vi "Load Config.vi"(11 "Config Path":path) -> (1 "Twitter":cluster{"Enabled":bool, "Tag":string}, 2 "Flickr":T2, 3 "Photobooth":T1)   [LabVIEW 2012]
uses:
  <vilib>/Utility/config.llb/NI_LVConfig.lvlib
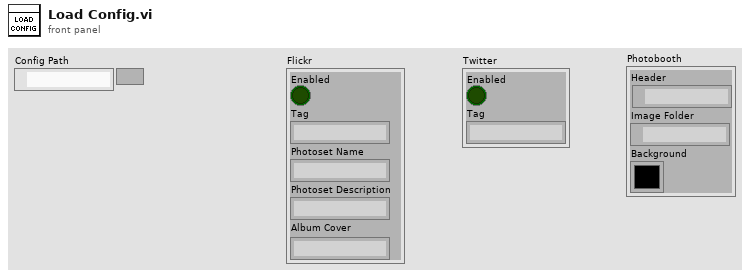
[diagram p1: front panel]
types:
  T1 = cluster{"Header":path, "Image Folder":path, "Background":u32}
  T2 = cluster{"Enabled":bool, "Tag":string, "Photoset Name":string, "Photoset Description":string, "Album Cover":string}
  T3 = cluster{"Header":path, "Image Folder":path, "Background":cluster{"Red":u8, "Green":u8, "Blue":u8}}
  T4 = typedef "NI_LVConfig.lvlib/Config Data RefNum.ctl" = refnum<k1>
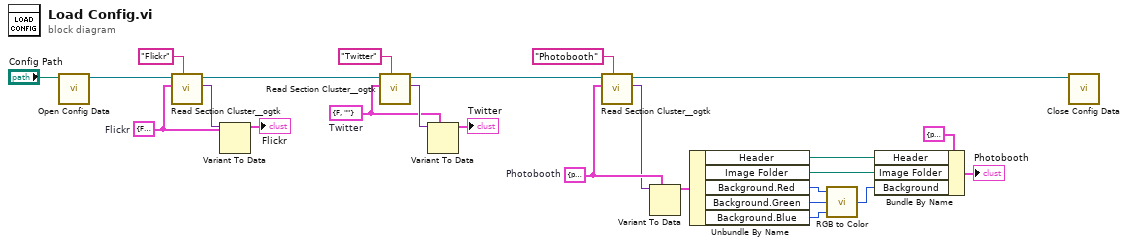
[diagram p0: block diagram]
diagram:
  w14 = T3 {"Header"=path "", "Image Folder"=path "", "Background"={"Red"=0, "Green"=0, "Blue"=0}}  # Photobooth
  w15 = cluster{"Enabled":bool, "Text":string} {"Enabled"=FALSE, "Text"=""}  # Twitter
  w22 = T2 {"Enabled"=FALSE, "Tag"="", "Photoset Name"="", "Photoset Description"="", "Album Cover"=""}  # Flickr
  n1 = call <vilib>:"Open Config Data.vi"("configuration file path"="Config Path") -> ("refnum"=w24:T4)  [unwired: 8 in, 2 out]
  n2 = call <userlib>:"Read Section Cluster__ogtk.vi"("section (optional)"="Flickr", "Section Formatted Cluster Type"=w22, "refnum"=w24) -> ("Section Formatted Cluster"=w20:variant, "dup refnum"=w16:T4)  [unwired: 4 in, 3 out]
  n3 = Variant To Data(type=w22, Variant=w20) -> (data=→"Flickr":T2)  [unwired: 1 in, 1 out]
  n4 = call <userlib>:"Read Section Cluster__ogtk.vi"("section (optional)"="Twitter", "Section Formatted Cluster Type"=w15, "refnum"=w16) -> ("Section Formatted Cluster"=w19:variant, "dup refnum"=w11:T4)  [unwired: 4 in, 3 out]
  n5 = Variant To Data(type=w15, Variant=w19) -> (data=→"Twitter":cluster{"Enabled":bool, "Text":string})  [unwired: 1 in, 1 out]
  n6 = call <userlib>:"Read Section Cluster__ogtk.vi"("section (optional)"="Photobooth", "Section Formatted Cluster Type"=w14, "refnum"=w11) -> ("Section Formatted Cluster"=w12:variant, "dup refnum"=w10:T4)  [unwired: 4 in, 3 out]
  n7 = Variant To Data(type=w14, Variant=w12) -> (data=w9:T3)  [unwired: 1 in, 1 out]
  n8 = Unbundle By Name(w9) -> ("Header"=w2:path, "Image Folder"=w1:path, "Background.Red"=w6:u8, "Background.Green"=w5:u8, "Background.Blue"=w4:u8)
  n9 = call <vilib>:"RGB to Color.vi"("B"=w4, "G"=w5, "R"=w6) -> ("Color"=w3:u32)
  n10 = Bundle By Name(cluster=T1 {"Header"=path "", "Image Folder"=path "", "Background"=0} ("Photobooth"), "Header"=w2, "Image Folder"=w1, "Background"=w3) -> (→"Photobooth":T1)
  n11 = call <vilib>:"Close Config Data.vi"("refnum"=w10) -> ()  [unwired: 9 in, 2 out]
